vi "Core.vi"(0 "A":bool, 1 "Parameters":T2, 5 "B":bool, 7 "Z":bool, 11 "reset":bool) -> (4 "Output":T1, 6 "CW_direction":bool, 10 "AbsPosition":i32, 15 "RevPosition":i32)   [LabVIEW 2015, in "QuadEnc.lvlib"]
uses:
  QuadEnc.lvlib
  Parameters.ctl
  Output.ctl
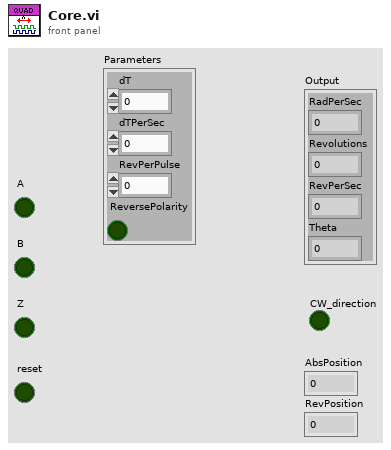
[diagram p1: front panel]
types:
  T1 = typedef "QuadEnc.lvlib/Output.ctl" = cluster{"RadPerSec":sgl, "Revolutions":sgl, "RevPerSec":sgl, "Theta":sgl}
  T2 = typedef "QuadEnc.lvlib/Parameters.ctl" = cluster{"dT":u32, "dTPerSec":sgl, "RevPerPulse":sgl, "ReversePolarity":bool}
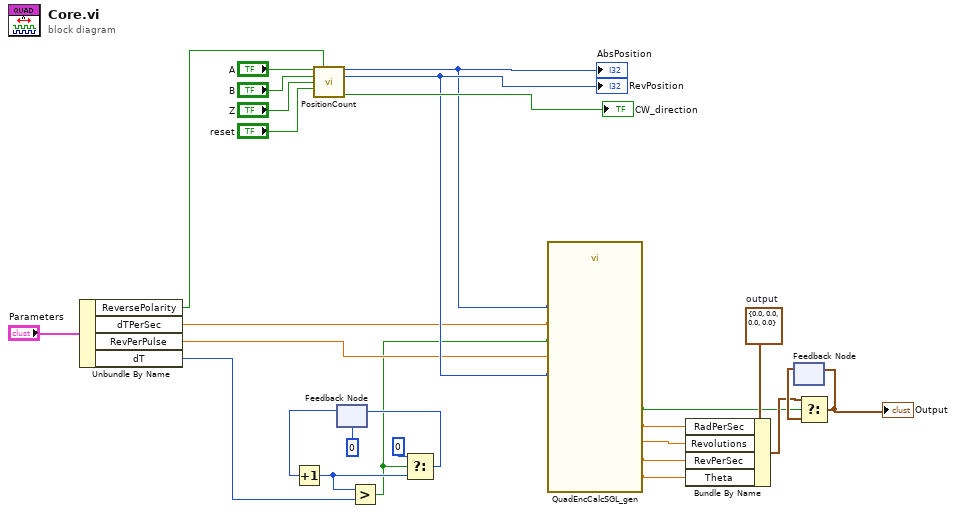
[diagram p0: block diagram]
diagram:
  w19 = T1 {"RadPerSec"=0.0, "Revolutions"=0.0, "RevPerSec"=0.0, "Theta"=0.0}  # output
  n1 = Unbundle By Name("Parameters") -> ("ReversePolarity"=w17:bool, "dTPerSec"=w3:sgl, "RevPerPulse"=w4:sgl, "dT"=w14:u32)
  n2 = call "PositionCount.vi"("A"="A", "ReversePolarity"=w17, "B"="B", "Z"="Z", "reset"="reset") -> ("AbsPosition"=w2:i32, "RevPosition"=w5:i32, "CW_direction"=→"CW_direction":bool)  [unwired: 8 in]
  "AbsPosition" <- w2
  "RevPosition" <- w5
  n3 = feedback #1(u32 0 ("dT")) -> (w16:u32)
  n4 = Increment(x=w16) -> (x+1=w13:u32)
  n5 = Greater?(x=w13, y=w14) -> (0:w1:bool)
  n6 = Select(t=u32 0, s=w1, f=w13) -> (s? t:f=w12:u32)
  n7 = feedback-in #1(w12) -> ()
  n8 = call "QuadEncCalcSGL_gen.vi"("AbsPosition"=w2, "RevPosition"=w5, "input valid"=w1, "RevPerPulse"=w4, "dTPerSec"=w3) -> ("Revolutions"=w9:sgl, "RevPerSec"=w8:sgl, "Theta"=w7:sgl, "output valid"=w6:bool, "RadPerSec"=w10:sgl)  [unwired: 5 in, 1 out]
  n9 = Bundle By Name(cluster=w19, "RadPerSec"=w10, "Revolutions"=w9, "RevPerSec"=w8, "Theta"=w7) -> (w18:T1)
  n10 = feedback #2() -> (w21:T1)  [unwired: 1 in]
  n11 = Select(t=w18, s=w6, f=w21) -> (s? t:f=w20:T1)
  "Output" <- w20
  n12 = feedback-in #2(w20) -> ()
